vi "PID_calc_AmplitudeFeedback_test_C.vi"(4 "Kd/Tau":fxp<+/-,32,6>, 5 "Ki*Tau":fxp<+/-,32,6>, 6 "Kp":fxp<+/-,32,6>, 7 "Enabled":bool=TRUE, 8 "input valid":bool=TRUE, 11 "Data in":fxp<+/-,16,14>[](array[numeric])=[0.0, 0.0, 0.0, 0.0]) -> (0 "output valid":bool, 1 "c(t) valid":bool, 2 "c(t)":fxp<+/-,32,21>, 3 "data out":fxp<+/-,16,14>[](array[numeric]))   [LabVIEW 2013]
uses:
  <vilib>/rvi/FXPMathLib/FxpDiv/subVIs/nifxpmath_Div_SimConfig.ctl
  <vilib>/rvi/FXPMathLib/FxpDiv/simVIs/DllFxpDivTemp_sub.vi
  <vilib>/rvi/FXPMathLib/FxpDiv/XNode/nifxpmath_Div.xnode
  <vilib>/rvi/FXPMathLib/FxpSub/XNode/nifxpmath_Sub.xnode
  <vilib>/rvi/FXPMathLib/FxpMul/XNode/nifxpmath_Multiplier.xnode
  <vilib>/rvi/FXPMathLib/FxpAdd/XNode/nifxpmath_Add.xnode
  <vilib>/rvi/FXPMathLib/sim/FxpSim.dll
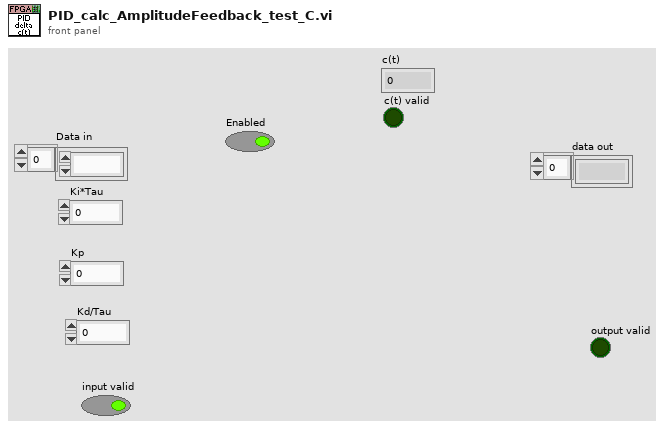
[diagram p1: front panel]
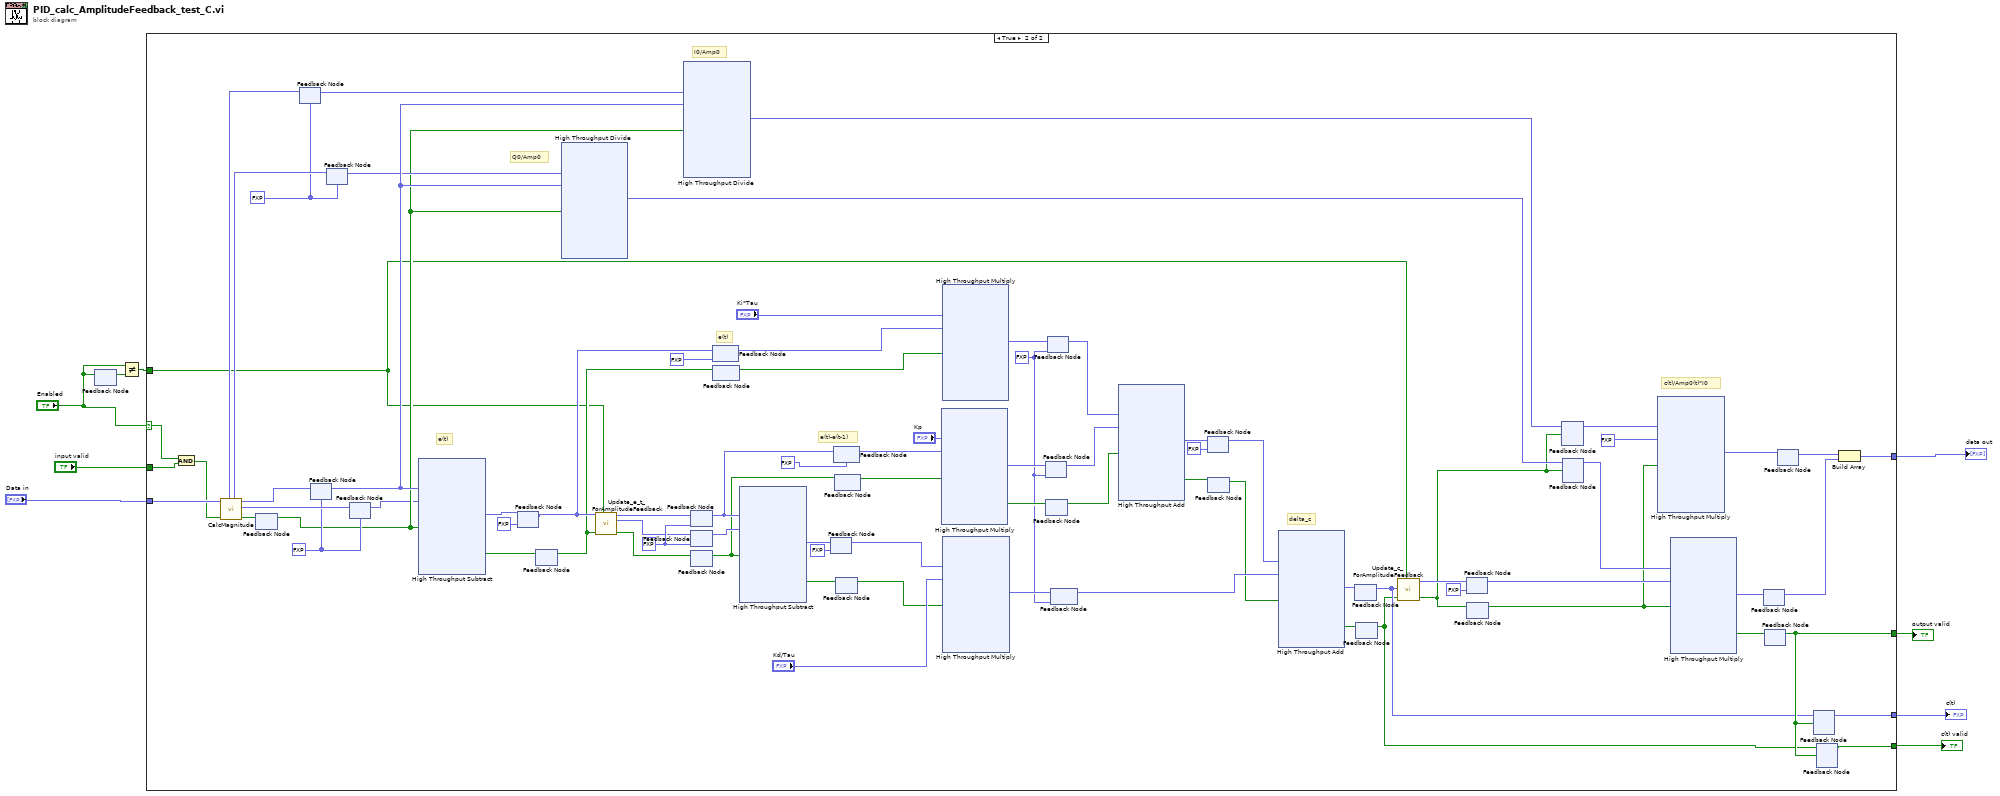
[diagram p0: block diagram]
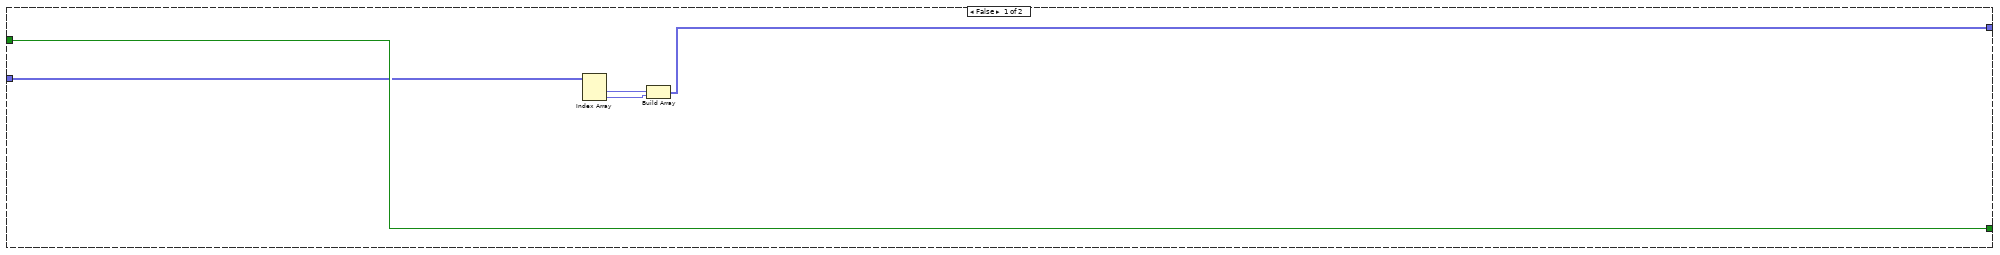
[diagram p2: hidden frame]
diagram:
  n1 = feedback #1() -> (w3:bool)  [unwired: 1 in]
  n2 = feedback-in #1("Enabled") -> ()
  n3 = Not Equal?(x="Enabled", y=w3) -> (x != y?=w1:bool)
  n4 = case shown="True" "Enabled" {
    selector: "Enabled" -> [_ w24]
    tunnel: "Data in" -> [w13 w72]
    tunnel: [w14 w18] -> w8
    tunnel: [w10 w52] -> w7
    tunnel: "input valid" -> [w14 w34]
    tunnel: [_ w21] -> w5
    tunnel: [_ w20] -> w4
    tunnel: w1 -> [_ w23]
    frame False {
      n5 = Index Array(array=w13) -> (element #1=w12:fxp<+/-,16,14>, element #2=w11:fxp<+/-,16,14>)  [unwired: 2 in]
      n6 = Build Array(w12, w11) -> (w10:fxp<+/-,16,14>[])
    }
    frame True {
      w73 = fxp<+/-,32,21> 0.0 ("x*y")
      w50 = fxp<+/-,18,16> 0.0 ("e(t-1)-e(t-2)")
      w62 = fxp<+/-,16,14> 0.0 ("Q0 in")
      w68 = fxp<+,16,14> 0.0 ("Amp0")
      # "c(t)/Amp0(t)*I0"
      # "Q0/Amp0"
      # "I0/Amp0"
      # "delta_c"
      # "e(t)-e(t-1)"
      # "e(t)"
      # "e(t)"
      n7 = And(x=w24, y=w34) -> (x .and. y?=w33:bool)
      n8 = call "CalcMagnitude.vi"("input valid"=w33, "Data in"=w72) -> ("output valid"=w69:bool, "Amp1"=w70:fxp<+,16,14>, "Amp0"=w71:fxp<+,16,14>, "Q0 in"=w64:fxp<+/-,16,14>, "I0 in"=w66:fxp<+/-,16,14>)  [unwired: 5 in]
      n9 = feedback #2() -> (w43:bool)  [unwired: 1 in]
      n10 = feedback-in #2(w69) -> ()
      n11 = feedback #3(w62) -> (w65:fxp<+/-,16,14>)
      n12 = feedback-in #3(w66) -> ()
      n13 = feedback #4(w68) -> (w67:fxp<+,16,14>)
      n14 = feedback-in #4(w71) -> ()
      n15 = feedback #5(w62) -> (w63:fxp<+/-,16,14>)
      n16 = feedback-in #5(w64) -> ()
      n17 = feedback #6(w68) -> (w42:fxp<+,16,14>)
      n18 = feedback-in #6(w70) -> ()
      n19 = xnode "High Throughput Subtract"("x"=w67, "y"=w42, "input valid"=w43) -> ("x-y"=w40:fxp<+/-,17,15>, "output valid"=w41:bool)  [unwired: 1 in, 1 out]
      n20 = feedback #7(fxp<+/-,17,15> 0.0 ("x-y")) -> (w26:fxp<+/-,17,15>)
      n21 = feedback-in #7(w40) -> ()
      n22 = feedback #8() -> (w25:bool)  [unwired: 1 in]
      n23 = feedback-in #8(w41) -> ()
      n24 = xnode "High Throughput Divide"("x"=w63, "y"=w67, "input valid"=w43) -> ("x/y"=w59:fxp<+/-,32,16>)  [unwired: 1 in, 2 out]
      n25 = call "Update_e_t_ForAmplitudeFeedback.vi"("Rest"=w23, "input valid"=w25, "e(t)"=w26) -> ("output valid"=w29:bool, "e(t-1)-e(t-2)"=w35:fxp<+/-,18,16>, "e(t)-e(t-1)"=w30:fxp<+/-,18,16>)  [unwired: 6 in]
      n26 = xnode "High Throughput Divide"("x"=w65, "y"=w67, "input valid"=w43) -> ("x/y"=w61:fxp<+/-,32,16>)  [unwired: 1 in, 2 out]
      n27 = feedback #9(w50) -> (w75:fxp<+/-,18,16>)
      n28 = feedback-in #9(w30) -> ()
      n29 = feedback #10(w50) -> (w94:fxp<+/-,18,16>)
      n30 = feedback-in #10(w35) -> ()
      n31 = feedback #11() -> (w74:bool)  [unwired: 1 in]
      n32 = feedback-in #11(w29) -> ()
      n33 = feedback #12(fxp<+/-,17,15> 0.0 ("x-y")) -> (w88:fxp<+/-,17,15>)
      n34 = feedback-in #12(w26) -> ()
      n35 = feedback #13() -> (w86:bool)  [unwired: 1 in]
      n36 = feedback-in #13(w25) -> ()
      n37 = xnode "High Throughput Subtract"("x"=w75, "y"=w94, "input valid"=w74) -> ("x-y"=w92:fxp<+/-,19,17>, "output valid"=w91:bool)  [unwired: 1 in, 1 out]
      n38 = feedback #14(fxp<+/-,19,17> 0.0 ("x-y")) -> (w90:fxp<+/-,19,17>)
      n39 = feedback-in #14(w92) -> ()
      n40 = feedback #15(fxp<+/-,18,16> 0.0 ("e(t-1)-e(t-2)")) -> (w32:fxp<+/-,18,16>)
      n41 = feedback-in #15(w75) -> ()
      n42 = feedback #16() -> (w31:bool)  [unwired: 1 in]
      n43 = feedback-in #16(w74) -> ()
      n44 = feedback #17() -> (w87:bool)  [unwired: 1 in]
      n45 = feedback-in #17(w91) -> ()
      n46 = xnode ("High Throughput Multiply")("x"="Kp", "y"=w32, "input valid"=w31) -> ("x*y"=w83:fxp<+/-,32,21>, "output valid"=w82:bool)  [unwired: 1 in, 1 out]
      n47 = xnode ("High Throughput Multiply")("x"="Ki*Tau", "y"=w88, "input valid"=w86) -> ("x*y"=w85:fxp<+/-,32,21>)  [unwired: 1 in, 2 out]
      n48 = xnode ("High Throughput Multiply")("x"=w90, "y"="Kd/Tau", "input valid"=w87) -> ("x*y"=w81:fxp<+/-,32,21>)  [unwired: 1 in, 2 out]
      n49 = feedback #18(w73) -> (w28:fxp<+/-,32,21>)
      n50 = feedback-in #18(w83) -> ()
      n51 = feedback #19() -> (w27:bool)  [unwired: 1 in]
      n52 = feedback-in #19(w82) -> ()
      n53 = feedback #20(w73) -> (w84:fxp<+/-,32,21>)
      n54 = feedback-in #20(w85) -> ()
      n55 = feedback #21(w73) -> (w80:fxp<+/-,32,21>)
      n56 = feedback-in #21(w81) -> ()
      n57 = xnode "High Throughput Add"("x"=w84, "y"=w28, "input valid"=w27) -> ("x+y"=w79:fxp<+/-,32,21>, "output valid"=w78:bool)  [unwired: 1 in, 1 out]
      n58 = feedback #22(fxp<+/-,32,21> 0.0 ("x+y")) -> (w77:fxp<+/-,32,21>)
      n59 = feedback-in #22(w79) -> ()
      n60 = feedback #23() -> (w76:bool)  [unwired: 1 in]
      n61 = feedback-in #23(w78) -> ()
      n62 = xnode "High Throughput Add"("x"=w77, "y"=w80, "input valid"=w76) -> ("x+y"=w37:fxp<+/-,32,21>, "output valid"=w36:bool)  [unwired: 1 in, 1 out]
      n63 = feedback #24() -> (w17:fxp<+/-,32,21>)  [unwired: 1 in]
      n64 = feedback-in #24(w37) -> ()
      n65 = feedback #25() -> (w16:bool)  [unwired: 1 in]
      n66 = feedback-in #25(w36) -> ()
      n67 = call "Update_c_ForAmplitudeFeedback.vi"("Reset"=w23, "input valid"=w16, "delta_c"=w17) -> ("output valid"=w19:bool, "c out"=w22:fxp<+/-,32,21>)  [unwired: 7 in]
      n68 = feedback #26(fxp<+/-,32,21> 0.0 ("c out")) -> (w39:fxp<+/-,32,21>)
      n69 = feedback-in #26(w22) -> ()
      n70 = feedback #27() -> (w38:bool)  [unwired: 1 in]
      n71 = feedback-in #27(w19) -> ()
      n72 = feedback #28() -> (w60:fxp<+/-,32,16>)  [unwired: 1 in]
      n73 = feedback-in #28(w61, w19) -> ()
      n74 = feedback #29() -> (w58:fxp<+/-,32,16>)  [unwired: 1 in]
      n75 = feedback-in #29(w59, w19) -> ()
      n76 = xnode ("High Throughput Multiply")("x"=w60, "y"=fxp<+/-,32,21> 1.0, "input valid"=w38) -> ("x*y"=w57:fxp<+/-,16,14>)  [unwired: 1 in, 2 out]
      n77 = xnode ("High Throughput Multiply")("x"=w58, "y"=w39, "input valid"=w38) -> ("x*y"=w56:fxp<+/-,16,14>, "output valid"=w55:bool)  [unwired: 1 in, 1 out]
      n78 = feedback #30() -> (w53:fxp<+/-,16,14>)  [unwired: 1 in]
      n79 = feedback-in #30(w56) -> ()
      n80 = feedback #31() -> (w18:bool)  [unwired: 1 in]
      n81 = feedback-in #31(w55) -> ()
      n82 = feedback #32() -> (w54:fxp<+/-,16,14>)  [unwired: 1 in]
      n83 = feedback-in #32(w57) -> ()
      n84 = feedback #33() -> (w21:fxp<+/-,32,21>)  [unwired: 1 in]
      n85 = feedback-in #33(w17, w18) -> ()
      n86 = feedback #34() -> (w20:bool)  [unwired: 1 in]
      n87 = feedback-in #34(w16, w18) -> ()
      n88 = Build Array(w54, w53) -> (w52:fxp<+/-,16,14>[])
    }
  }
  "output valid" <- w8
  "data out" <- w7
  "c(t)" <- w5
  "c(t) valid" <- w4
